vi "Vision Code_4.vi"(0 "Image In":T1, 1 "Image Dst":T1, 2 "Final Image Output":T1, 7 "error in":errorcluster) -> (20 "Image Out":T1, 21 "Output Image":T1(plugin-control), 27 "error out":errorcluster)   [LabVIEW 2014]
doc: "Creates, edits, and runs vision algorithms using NI Vision Assistant.\n\nWhen you place this Express VI on the block diagram, NI Vision Assistant launches. Create an algorithm using the Vision Assistant processing functions. After you create an algorithm, you can select the controls and indicators that you want to be able to programmatically set in LabVIEW. Double-click the Vision Assistant Express VI to edit the algorithm."
uses:
  <vilib>/vision/Image Controls.llb/IMAQ Image.ctl
  <vilib>/vision/NI_Vision_Development_Module.lvlib
panel:
  out "Particle Measurements (Pixels)":dbl[][](array[numeric]) format="%.2f"
  out "Number of Particles":i32
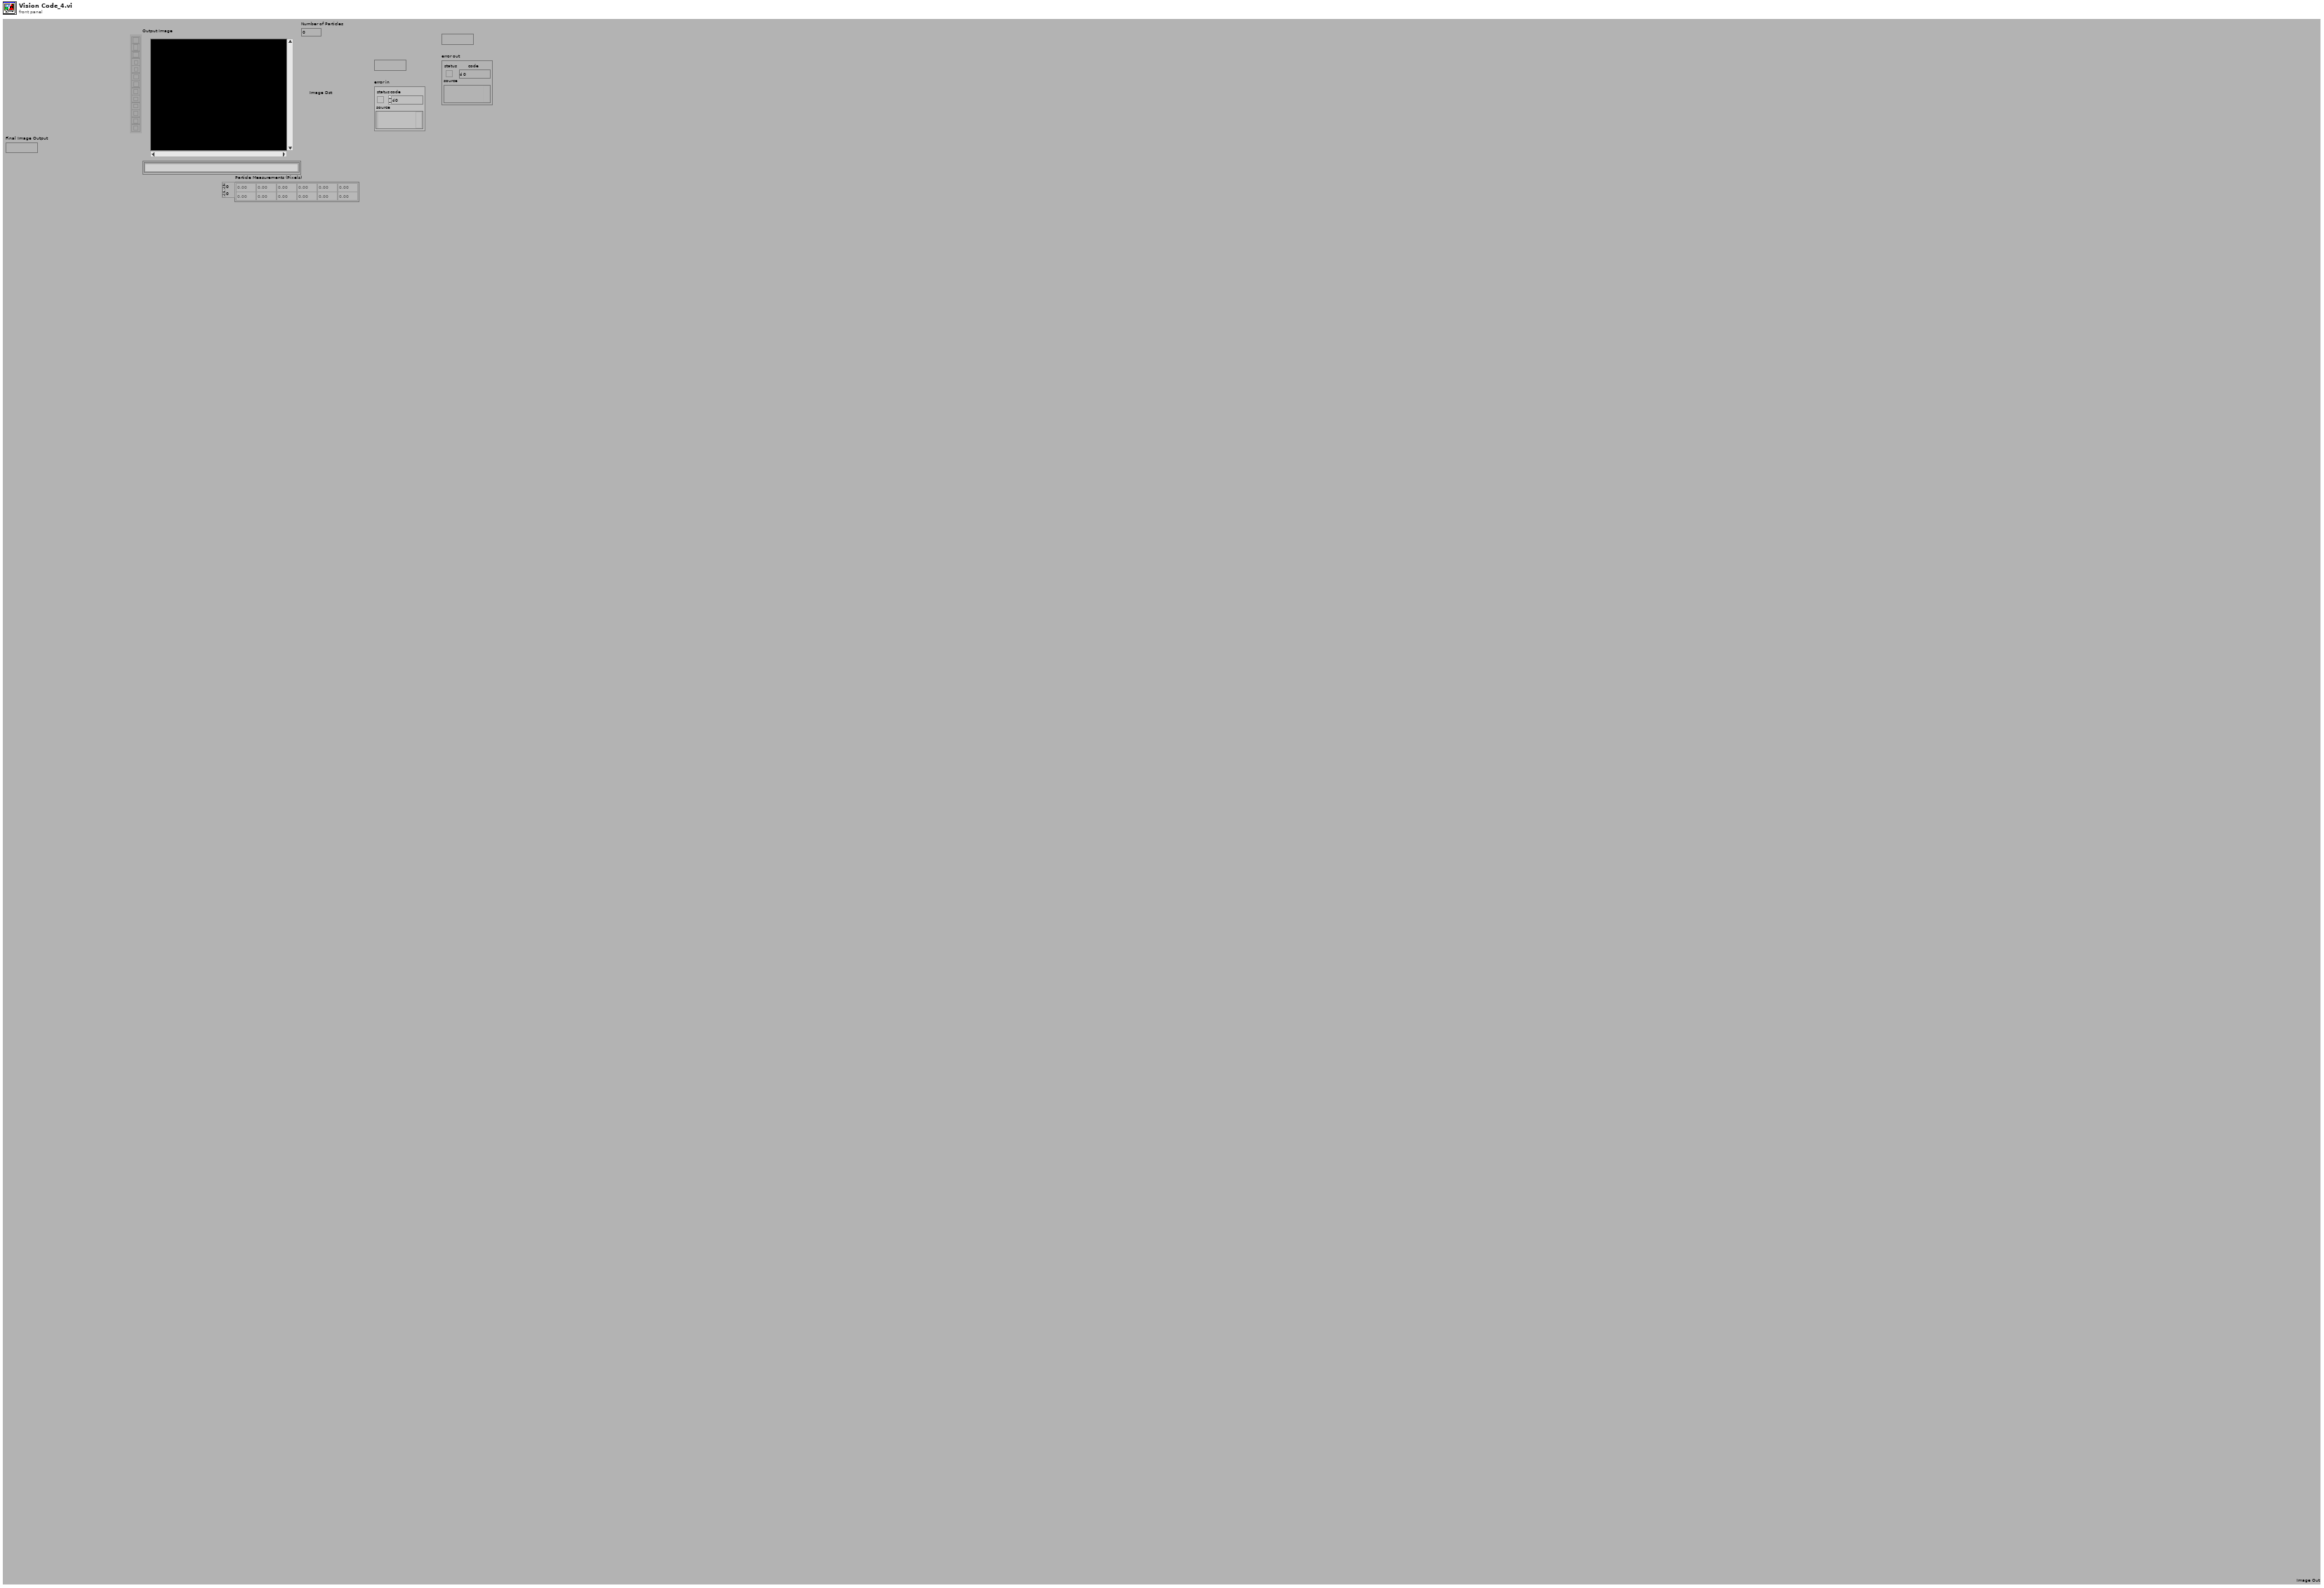
[diagram p1: front panel]
types:
  T1 = typedef "IMAQ Image.ctl" = refnum<image>
  T2 = cluster{"Global Rectangle":i32[], "Contours":cluster{"ID":enum32{"External", "Internal"}, "Type":u32, "Coordinates":i32[]}[]}
  T3 = typedef "Image Type" = u32
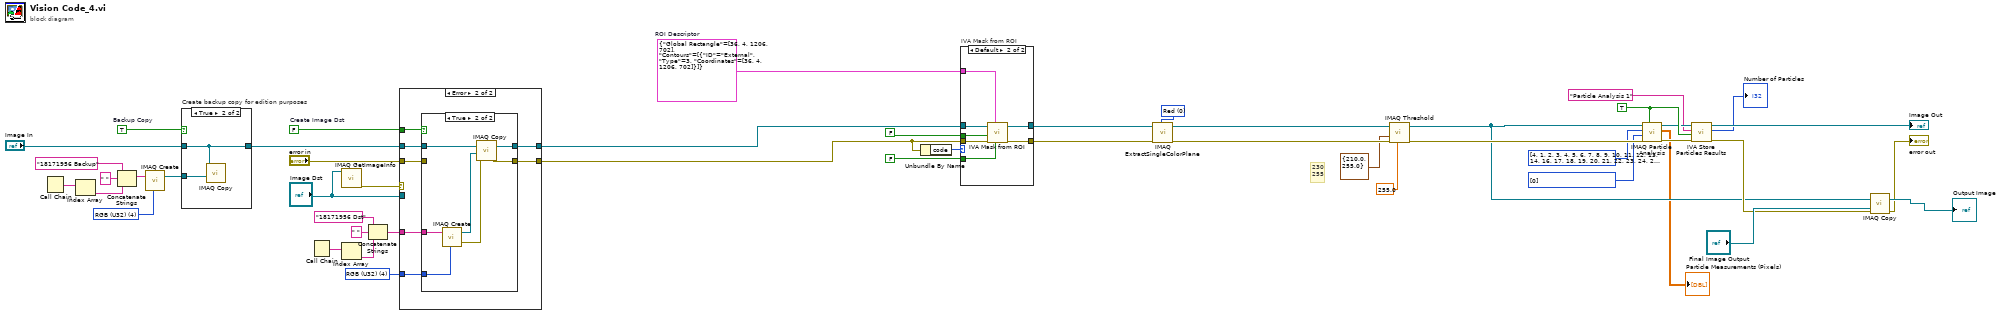
[diagram p0: block diagram]
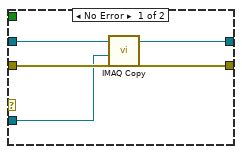
[diagram p3: hidden frame]
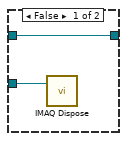
[diagram p5: hidden frame]
diagram:
  w14 = i32[] [0] items=["Center of Mass X", "Center of Mass Y", "First Pixel X", "First Pixel Y", "Bounding Rect Left", "Bounding Rect Top", "Bounding Rect Right", "Bounding Rect Bottom", "Max Feret Diameter Start X", "Max Feret Diameter Start Y", "Max Feret Diameter End X", "Max Feret Diameter End Y", "Max Horiz. Segment Length Left", "Max Horiz. Segment Length Right", "Max Horiz. Segment Length Row", "-", "Bounding Rect Width", "Bounding Rect Height", "Bounding Rect Diagonal", "Perimeter", "Convex Hull Perimeter", "Holes' Perimeter", "Max Feret Diameter", "Equivalent Ellipse Major Axis", "Equivalent Ellipse Minor Axis", "Equivalent Ellipse Minor Axis (Feret)", "Equivalent Rect Long Side", "Equivalent Rect Short Side", "Equivalent Rect Diagonal", "Equivalent Rect Short Side (Feret)", "Average Horiz. Segment Length", "Average Vert. Segment Length", "Hydraulic Radius", "Waddel Disk Diameter", "-", "Area", "Holes' Area", "Particle & Holes' Area", "Convex Hull Area", "Image Area", "-", "Number of Holes", "Number of Horiz. Segments", "Number of Vert. Segments", "-", "Orientation", "Max Feret Diameter Orientation", "-", "% Area/Image Area", "% Area/(Particle & Holes' Area)", "Ratio of Equivalent Ellipse Axes", "Ratio of Equivalent Rect Sides", "-", "Elongation Factor", "Compactness Factor", "Heywood Circularity Factor", "Type Factor", "-", "Sum X", "Sum Y", "Sum XX", "Sum XY", "Sum YY", "Sum XXX", "Sum XXY", "Sum XYY", "Sum YYY", "-", "Moment of Inertia XX", "Moment of Inertia XY", "Moment of Inertia YY", "Moment of Inertia XXX", "Moment of Inertia XXY", "Moment of Inertia XYY", "Moment of Inertia YYY", "Norm. Moment of Inertia XX", "Norm. Moment of Inertia XY", "Norm. Moment of Inertia YY", "Norm. Moment of Inertia XXX", "Norm. Moment of Inertia XXY", "Norm. Moment of Inertia XYY", "Norm. Moment of Inertia YYY", "Hu Moment 1", "Hu Moment 2", "Hu Moment 3", "Hu Moment 4", "Hu Moment 5", "Hu Moment 6", "Hu Moment 7"] ("Real-World Measurements")
  w15 = i32[] [4, 1, 2, 3, 4, 5, 6, 7, 8, 9, 10, 11, 12, 13, 14, 16, 17, 18, 19, 20, 21, 22, 23, 24, 25, 26, 27, 28, 29, 30, 31, 32, 33, 35, 36, 37, 38, 39, 41, 42, 43, 45, 46, 48, 49, 50, 51, 53, 54, 55, 56, 58, 59, 60, 61, 62, 63, 64, 65, 66, 68, 69, 70, 71, 72, 73, 74, 75, 76, 77, 78, 79, 80, 81, 82, 83, 84, 85, 86, 87, 88] items=["Center of Mass X", "Center of Mass Y", "First Pixel X", "First Pixel Y", "Bounding Rect Left", "Bounding Rect Top", "Bounding Rect Right", "Bounding Rect Bottom", "Max Feret Diameter Start X", "Max Feret Diameter Start Y", "Max Feret Diameter End X", "Max Feret Diameter End Y", "Max Horiz. Segment Length Left", "Max Horiz. Segment Length Right", "Max Horiz. Segment Length Row", "-", "Bounding Rect Width", "Bounding Rect Height", "Bounding Rect Diagonal", "Perimeter", "Convex Hull Perimeter", "Holes' Perimeter", "Max Feret Diameter", "Equivalent Ellipse Major Axis", "Equivalent Ellipse Minor Axis", "Equivalent Ellipse Minor Axis (Feret)", "Equivalent Rect Long Side", "Equivalent Rect Short Side", "Equivalent Rect Diagonal", "Equivalent Rect Short Side (Feret)", "Average Horiz. Segment Length", "Average Vert. Segment Length", "Hydraulic Radius", "Waddel Disk Diameter", "-", "Area", "Holes' Area", "Particle & Holes' Area", "Convex Hull Area", "Image Area", "-", "Number of Holes", "Number of Horiz. Segments", "Number of Vert. Segments", "-", "Orientation", "Max Feret Diameter Orientation", "-", "% Area/Image Area", "% Area/(Particle & Holes' Area)", "Ratio of Equivalent Ellipse Axes", "Ratio of Equivalent Rect Sides", "-", "Elongation Factor", "Compactness Factor", "Heywood Circularity Factor", "Type Factor", "-", "Sum X", "Sum Y", "Sum XX", "Sum XY", "Sum YY", "Sum XXX", "Sum XXY", "Sum XYY", "Sum YYY", "-", "Moment of Inertia XX", "Moment of Inertia XY", "Moment of Inertia YY", "Moment of Inertia XXX", "Moment of Inertia XXY", "Moment of Inertia XYY", "Moment of Inertia YYY", "Norm. Moment of Inertia XX", "Norm. Moment of Inertia XY", "Norm. Moment of Inertia YY", "Norm. Moment of Inertia XXX", "Norm. Moment of Inertia XXY", "Norm. Moment of Inertia XYY", "Norm. Moment of Inertia YYY", "Hu Moment 1", "Hu Moment 2", "Hu Moment 3", "Hu Moment 4", "Hu Moment 5", "Hu Moment 6", "Hu Moment 7"] ("Pixel Measurements")
  w13 = TRUE ("Connectivity 4/8 (8)")
  w21 = 0 items=["Red", "Green", "Blue", "Hue", "Saturation", "Luminance", "Value", "Intensity"] ("Color Plane")
  w27 = T2 {"Global Rectangle"=[36, 4, 1206, 702], "Contours"=[{"ID"=enum."External", "Type"=3, "Coordinates"=[36, 4, 1206, 702]}]}  # ROI Descriptor
  w28 = T3 4 items=["Grayscale (U8)", "Grayscale (I16)", "Grayscale (SGL)", "Complex (CSG)", "RGB (U32)", "HSL (U32)", "RGB (U64)", "Grayscale (U16)"] ("Image Dst Type")
  w29 = T3 4 items=["Grayscale (U8)", "Grayscale (I16)", "Grayscale (SGL)", "Complex (CSG)", "RGB (U32)", "HSL (U32)", "RGB (U64)", "Grayscale (U16)"] ("Image Type")
  w48 = TRUE  # Backup Copy
  w41 = FALSE  # Create Image Dst
  # "230\n255"
  n1 = Call Chain() -> (call chain=w35:string[])
  n2 = Index Array(array=w35) -> (element=w34:string)  [unwired: 1 in]
  n3 = Concatenate Strings("18171956 Backup" ("Backup Image Name"), " ", w34) -> (w31:string)
  n4 = call "IMAQ Create"("Image Name"=w31, "Image Type"=w29) -> ("New Image"=w30:T1)  [unwired: 2 in, 2 out]
  n5 = case "Create backup copy for edition purposes" shown="True" w48 {
    tunnel: [w50 w52] -> w44
    tunnel: "Image In" -> [w50 w52]
    tunnel: w30 -> [w49 w51]
    frame False {
      n6 = call "IMAQ Dispose"("Image"=w49) -> ()  [unwired: 2 in, 4 out]
    }
    frame True {
      n7 = call "IMAQ Copy"("Image Dst"=w51, "Image Src"=w52) -> ()  [unwired: 1 in, 5 out]
    }
  }
  n8 = Call Chain() -> (call chain=w40:string[])
  n9 = call "IMAQ GetImageInfo"("Image"="Image Dst") -> ("error out"=w46:errorcluster)  [unwired: 1 in, 9 out]
  n10 = Index Array(array=w40) -> (element=w38:string)  [unwired: 1 in]
  n11 = Concatenate Strings("18171956 Dst" ("Image Dst Name"), " ", w38) -> (w36:string)
  n12 = case shown="Error" w46 {
    tunnel: [w57 w61] -> w25
    tunnel: [w56 w60] -> w42
    tunnel: w44 -> [w55 w62]
    tunnel: "error in" -> [w54 w58]
    tunnel: "Image Dst" -> [w53 _]
    tunnel: w36 -> [_ w64]
    tunnel: w28 -> [_ w63]
    tunnel: w41 -> [_ w59]
    frame No Error {
      n13 = call "IMAQ Copy"("error in (no error)"=w54, "Image Dst"=w53, "Image Src"=w55) -> ("error out"=w56:errorcluster, "Image Dst Out"=w57:T1)  [unwired: 3 out]
    }
    frame Error {
      n14 = case shown="True" w59 {
        tunnel: w64 -> [_ w73]
        tunnel: w63 -> [_ w72]
        tunnel: w62 -> [w66 w70]
        tunnel: [w66 w69] -> w61
        tunnel: [w65 w68] -> w60
        tunnel: w58 -> [w65 _]
        frame False {
        }
        frame True {
          n15 = call "IMAQ Create"("Image Name"=w73, "Image Type"=w72) -> ("New Image"=w71:T1, "error out"=w67:errorcluster)  [unwired: 2 in, 1 out]
          n16 = call "IMAQ Copy"("error in (no error)"=w67, "Image Dst"=w71, "Image Src"=w70) -> ("error out"=w68:errorcluster, "Image Dst Out"=w69:T1)  [unwired: 3 out]
        }
      }
    }
  }
  n17 = Unbundle By Name(w42) -> ("code"=w22:i32)
  n18 = case "IVA Mask from ROI" shown="Default" w22 {
    tunnel: w27 -> [_ w81]
    tunnel: FALSE ("Shrink") -> [_ w80]
    tunnel: w25 -> [w74 w79]
    tunnel: w42 -> [_ w78]
    tunnel: [_ w77] -> w24
    tunnel: [w74 w76] -> w20
    tunnel: FALSE ("Out / In") -> [_ w75]
    frame -1074396199, -1074396198 {
      # "Discard\nCoordinate\nSystem\nError"
    }
    frame Default {
      n19 = call <vilib>:"IVA Mask from ROI.vi"("Shrink"=w80, "ROI Descriptor"=w81, "error in (no error)"=w78, "Out / In"=w75, "Image Src"=w79) -> ("error out"=w77:errorcluster, "Image Out"=w76:T1)  [unwired: 5 out]
    }
  }
  n20 = call "IMAQ ExtractSingleColorPlane"("Color Plane"=w21, "error in (no error)"=w24, "Image Src"=w20) -> ("error out"=w19:errorcluster, "Image Dst Out"=w17:T1)  [unwired: 1 in, 6 out]
  n21 = call "IMAQ Threshold"("Replace Value"=sgl 255.0, "error in (no error)"=w19, "Range"=cluster{"Lower value":sgl, "Upper value":sgl} {"Lower value"=210.0, "Upper value"=255.0}, "Image Src"=w17) -> ("error out"=w16:errorcluster, "Image Dst Out"=w4:T1)  [unwired: 2 in, 4 out]
  n22 = call "IMAQ Particle Analysis"("Connectivity 4/8 (8)"=w13, "error in (no error)"=w16, "Real-World Measurements"=w14, "Pixel Measurements"=w15, "Image"=w4) -> ("error out"=w10:errorcluster, "Particle Measurements (Pixels)"=→"Particle Measurements (Pixels)":dbl[][], "Image Out (duplicate)"=w12:T1)  [unwired: 4 out]
  n23 = call <vilib>:"IVA Store Particles Results.vi"("error in (no error)"=w10, "Connectivity 4/8 (8)"=w13, "Step Name"="Particle Analysis 1", "Image in"=w12) -> ("error out"=w7:errorcluster, "Number of Particles"=→"Number of Particles":i32, "Image dup"=→"Image Out":T1)  [unwired: 5 out]
  n24 = call "IMAQ Copy"("error in (no error)"=w7, "Image Dst"="Final Image Output", "Image Src"=w4) -> ("error out"=→"error out":errorcluster, "Image Dst Out"=→"Output Image":T1)  [unwired: 3 out]
